vi "Demo_Andon get max ID_NOK.vi"(8 "error in (no error)":errorcluster, 10 "Station No.":string, 11 "Refnum in":T1) -> (0 "error out":errorcluster, 1 "TABLE NAME":string, 2 "MAX BREAKDOWN ID":i32, 3 "Refnum out":T1, 4 "REJECTION COUNT":i32)   [LabVIEW 2017]
uses:
  <vilib>/addons/database/Connection.llb/Conn ObjectReference.ctl
  <vilib>/addons/database/Connection.llb/Conn Execute.vi
  <vilib>/addons/database/Recordset.llb/Rec Fetch Recordset Data (R).vi
  <vilib>/addons/database/Recordset.llb/Rec Destroy - Connection.vi
  <vilib>/addons/database/NI_Database_API.lvlib
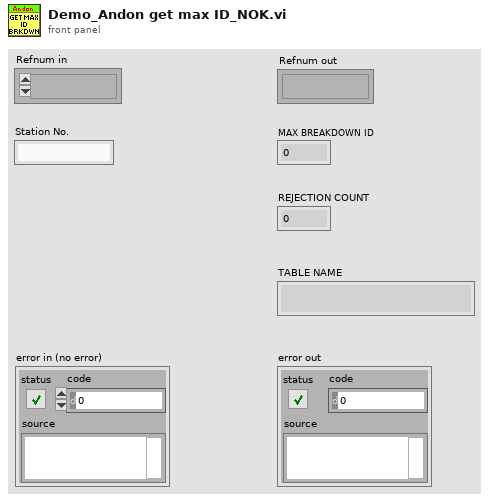
[diagram p1: front panel]
types:
  T1 = typedef "NI_Database_API.lvlib/Conn ObjectReference.ctl" = refnum<k1>
  T2 = typedef "NI_Database_API.lvlib/Rec ObjectReference.ctl" = refnum<k1>
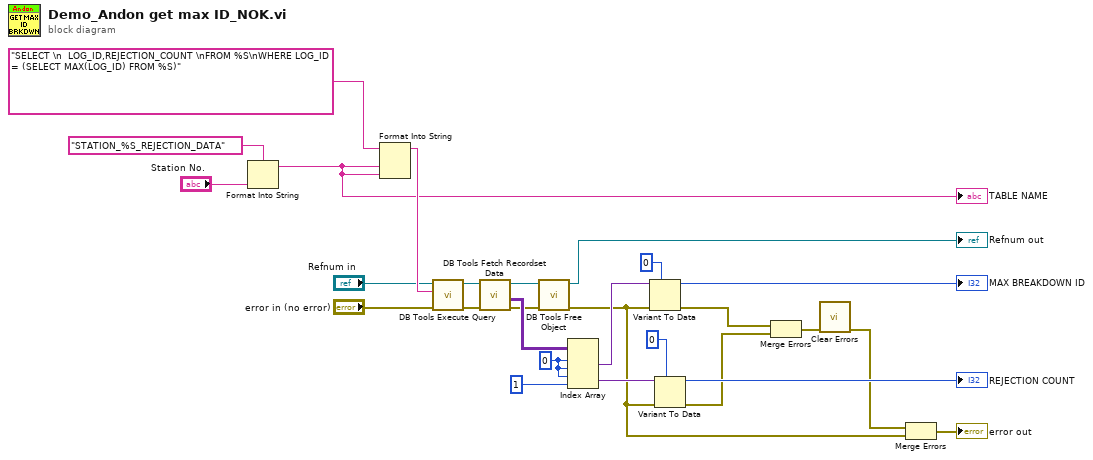
[diagram p0: block diagram]
diagram:
  w11 = 0 ("index (row)")
  n1 = Format Into String(format string="STATION_%S_REJECTION_DATA" ("SQL query"), "Station No.") -> (resulting string=w14:string)  [unwired: 2 in, 1 out]
  "TABLE NAME" <- w14
  n2 = Format Into String(format string="SELECT \n  LOG_ID,REJECTION_COUNT \nFROM %S\nWHERE LOG_ID = (SELECT MAX(LOG_ID) FROM %S)" ("SQL query"), w14, w14) -> (resulting string=w18:string)  [unwired: 2 in, 1 out]
  n3 = call-poly <vilib>:"DB Tools Execute Query.vi"("error in (no error)"="error in (no error)", "SQL query"=w18, "connection reference"="Refnum in") -> ("error out"=w22:errorcluster, "recordset reference"=w23:T2)  [unwired: 5 in]
  n4 = call-poly <vilib>:"DB Tools Fetch Recordset Data.vi"("error in (no error)"=w22, "recordset reference"=w23) -> ("error out"=w21:errorcluster, "recordset data"=w25:variant[][], "recordset reference out"=w24:T2)  [unwired: 3 in]
  n5 = call-poly <vilib>:"DB Tools Free Object.vi"("error in (no error)"=w21, "recordset reference"=w24) -> ("error out"=w2:errorcluster, "connection reference"=→"Refnum out":T1)  [unwired: 8 in]
  n6 = Index Array(array=w25, index (row) #1=w11, index (col) #1=w11, index (row) #2=w11, index (col) #2=1 ("index (row)")) -> (element #1=w19:variant, element #2=w10:variant)
  n7 = Variant To Data(error in=w2, type=0, Variant=w19) -> (data=→"MAX BREAKDOWN ID":i32, error out=w27:errorcluster)
  n8 = Variant To Data(error in=w2, type=0, Variant=w10) -> (data=→"REJECTION COUNT":i32, error out=w4:errorcluster)
  n9 = Merge Errors(w27, w4) -> (w5:errorcluster)
  n10 = call <vilib>:"Clear Errors.vi"("error in (no error)"=w5) -> ("error out"=w3:errorcluster)  [unwired: 5 in, 1 out]
  n11 = Merge Errors(w3, w2) -> (→"error out":errorcluster)
